vi "trio_getvr.vi"(6 "Error/Warning (Error)":bool, 8 "error in (no error)":errorcluster, 10 "Vr #":i16, 11 "reference in":refnum<k7>) -> (0 "error out":errorcluster, 2 "Value":dbl, 3 "reference out":refnum<k7>, 5 "GetVr":bool)   [LabVIEW 2024]
uses:
  <instrlib>/Trio Motion/Trio Motion Library.lvlib
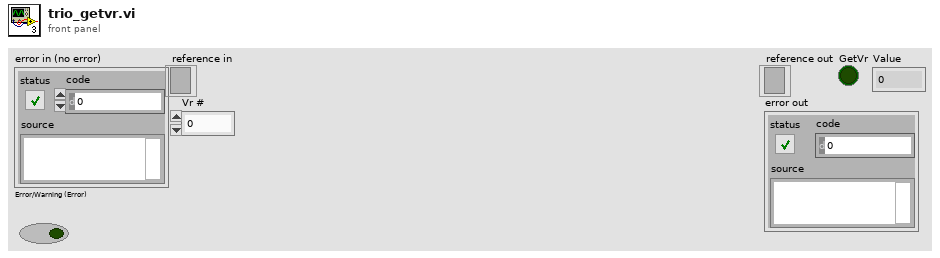
[diagram p1: front panel]
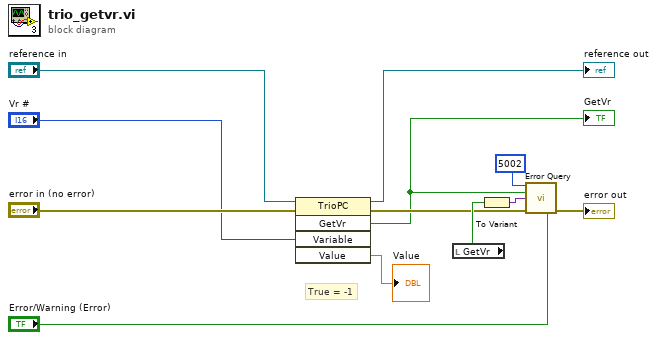
[diagram p0: block diagram]
diagram:
  # "True = -1"
  n1 = invoke class="TrioPC" method="GetVr"(reference="reference in", error in="error in (no error)", "Variable"="Vr #") -> (reference out=→"reference out":refnum<k7>, error out=w5:errorcluster, "GetVr"=w3:bool, "Value"=→"Value":dbl)  [unwired: 2 in, 1 out]
  "GetVr" <- w3
  n2 = local read "GetVr"() -> (w7:bool)
  n3 = To Variant(anything=w7) -> (Variant=w6:variant)
  n4 = call <instrlib>:"Error Query.vi"("error code (0)"=5002, "State"=w3, "Command"=w6, "error in (no error)"=w5, "Error/Warning (Error)"="Error/Warning (Error)") -> ("error out"=→"error out":errorcluster)  [unwired: 10 in]
